vi "UART_WR.vi"(0 "coms":refnum<visa-resource-name>, 1 "timeOut_s":dbl=1.8, 7 "hexSend":string, 11 "rdMatch":string, 12 "strType":enum16{"normal", "Hex"}(ring)=enum."Hex") -> (3 "log":string, 4 "data":string, 8 "Read":string, 15 "OK":bool)   [LabVIEW 2015]
uses:
  <vilib>/Instr/_visa.llb/VISA Configure Serial Port (Instr).vi
panel:
  out "time_ms":u32
  out "r":string
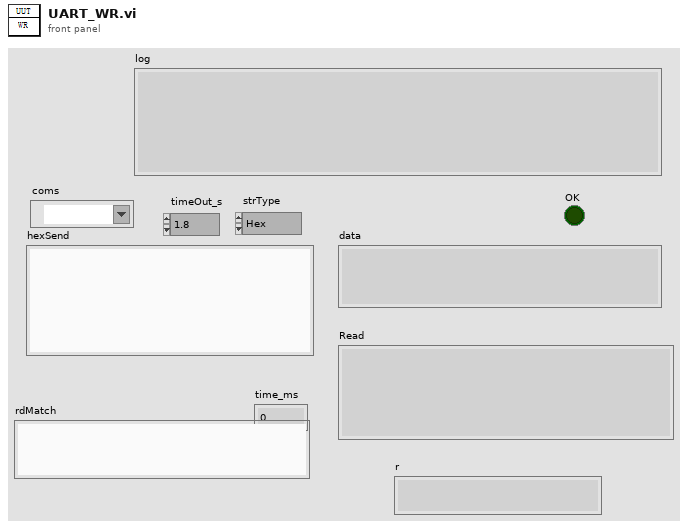
[diagram p1: front panel]
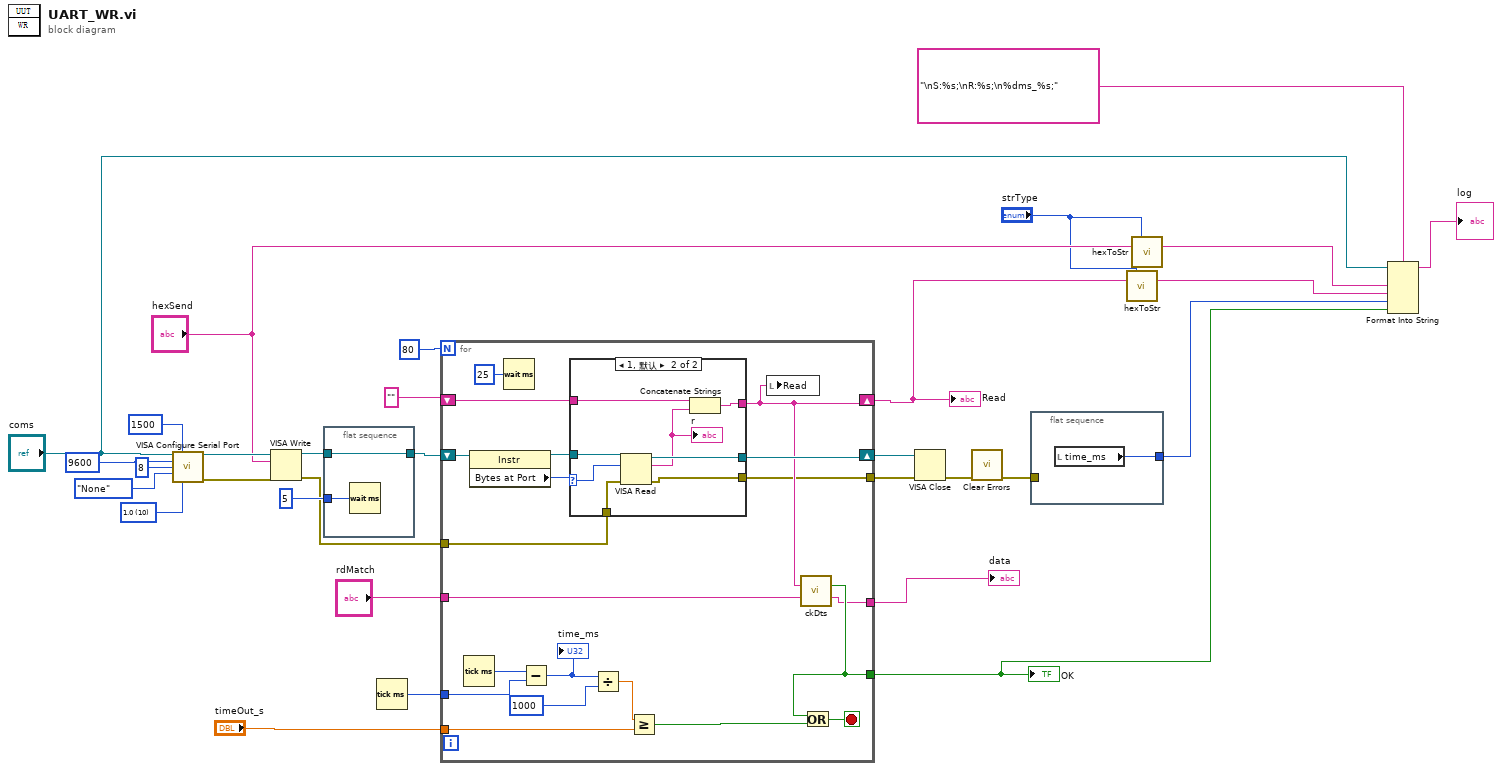
[diagram p0: block diagram]
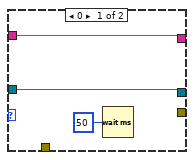
[diagram p2: hidden frame]
diagram:
  w27 = u16 10 items=["1.0"=10, "1.5"=15, "2.0"=20] ("stop bits (10: 1 bit)")
  n1 = call-poly "VISA Configure Serial Port"("VISA resource name"="coms", "timeout (10sec)"=u32 1500, "baud rate (9600)"=u32 9600, "data bits (8)"=u16 8, "parity (0:none)"=enum16{"None", "Odd", "Even", "Mark", "Space"}."None", "stop bits (10: 1 bit)"=w27) -> ("VISA resource name out"=w26:refnum<visa-resource-name>, "error out"=w3:errorcluster)  [unwired: 8 in]
  n2 = VISA Write(VISA resource name=w26, write buffer="hexSend", error in (no error)=w3) -> (VISA resource name out=w25:refnum<visa-resource-name>, error out=w2:errorcluster)  [unwired: 1 out]
  n3 = flat-sequence {
    tunnel: w25 -> [w33]
    tunnel: [w33] -> w23
    tunnel: u32 5 ("等待时间（毫秒）") -> [w32]
    frame #0 {
      n4 = Wait (ms)(milliseconds to wait=w32) -> ()  [unwired: 1 out]
    }
  }
  n5 = Tick Count (ms)() -> (millisecond timer value=w19:u32)
  n6 = for {
    N: 80 -> [_]
    shift-right: [w50] -> w20
    shift-left: w23 -> [w53]
    shift-right: [w39] -> w10
    shift-left: "" -> [w48]
    tunnel: w19 -> [w46]
    tunnel: "timeOut_s" -> [w44]
    tunnel: [w37] -> w6
    tunnel: [w36] -> w5
    tunnel: "rdMatch" -> [w38]
    tunnel: w2 -> [w35]
    tunnel: [w34] -> w1
    stop <- w42 stop-if-true
    n7 = Tick Count (ms)() -> (millisecond timer value=w47:u32)
    n8 = property class="Instr"(reference=w53) -> (reference out=w51:refnum<visa-resource-name>, "Bytes at Port"=w52:u32)  [unwired: 1 in, 1 out]
    n9 = Wait (ms)(milliseconds to wait=u32 25 ("等待时间（毫秒）")) -> ()  [unwired: 1 out]
    n10 = Subtract(x=w47, y=w46) -> (x-y=w40:u32)
    "time_ms" <- w40
    n11 = case shown="1, 默认" w52 {
      selector: w52 -> [_ w63]
      tunnel: w51 -> [w56 w64]
      tunnel: [w56 w62] -> w50
      tunnel: w48 -> [w54 w61]
      tunnel: [w54 w59] -> w39
      tunnel: w35 -> [_ w58]
      tunnel: [_ w57] -> w34
      frame 0 {
        n12 = Wait (ms)(milliseconds to wait=u32 50 ("等待时间（毫秒）")) -> ()  [unwired: 1 out]
      }
      frame 1, Default {
        n13 = VISA Read(VISA resource name=w64, byte count=w63, error in (no error)=w58) -> (VISA resource name out=w62:refnum<visa-resource-name>, read buffer=w60:string, error out=w57:errorcluster)  [unwired: 1 out]
        "r" <- w60
        n14 = Concatenate Strings(w61, w60) -> (w59:string)
      }
    }
    n15 = Divide(x=w40, y=u32 1000) -> (x/y=w41:dbl)
    n16 = Greater Or Equal?(x=w41, y=w44) -> (x >= y?=w43:bool)
    n17 = local write "Read"(w39) -> ()
    n18 = call "ckDts.vi"("rdDts"=w39, "rdMatch"=w38) -> ("OK"=w37:bool, "dataOut"=w36:string)  [unwired: 12 in]
    n19 = Or(x=w37, y=w43) -> (x .or. y?=w42:bool)
  }
  "Read" <- w10
  "OK" <- w6
  "data" <- w5
  n20 = VISA Close(VISA resource name=w20, error in (no error)=w1) -> (error out=w15:errorcluster)
  n21 = call <vilib>:"Clear Errors.vi"("error in (no error)"=w15) -> ("error out"=w13:errorcluster)  [unwired: 5 in, 1 out]
  n22 = flat-sequence {
    tunnel: w13 -> [_]
    tunnel: [w65] -> w7
    frame #0 {
      n23 = local read "time_ms"() -> (w65:u32)
    }
  }
  n24 = call "hexToStr.vi"("strType"="strType", "str"=w10) -> ("strOut"=w8:string)  [unwired: 13 in]
  n25 = call "hexToStr.vi"("strType"="strType", "str"="hexSend") -> ("strOut"=w11:string)  [unwired: 13 in]
  n26 = Format Into String(format string="\nS:%s;\nR:%s;\n%dms_%s;" ("格式字符串"), initial string="coms", w11, w8, w7, w6) -> (resulting string=→"log":string)  [unwired: 1 in, 1 out]
